vi "ScurrDataOut.vi"(8 "error in (no error)":errorcluster, 10 "测试类型":string, 11 "通道":u16(ring) items=["直流CH1", "直流CH2", "直流CH3", "直流CH4", "直流CH5", "直流CH6", "直流CH7", "直流CH8", ""]) -> (0 "error out 2":errorcluster, 3 "表格控件":string[][](table))   [LabVIEW 2014]
uses:
  <vilib>/addons/database/Connection.llb/DB Tools Open Connec (String).vi
  <vilib>/addons/database/Connection.llb/Conn Execute.vi
  <vilib>/addons/database/Recordset.llb/Rec Fetch Recordset Data (R).vi
  <vilib>/addons/database/Recordset.llb/Rec Destroy - Connection.vi
  <vilib>/addons/database/_DB Variant To Data/Database Variant To Data.xnode
  <vilib>/addons/database/NI_Database_API.lvlib
panel:
  in  "测试类型":u16(ring) items=["温循", "高温老练", "常温拷机", "自定义测试", "单次测试", "自动测试"]
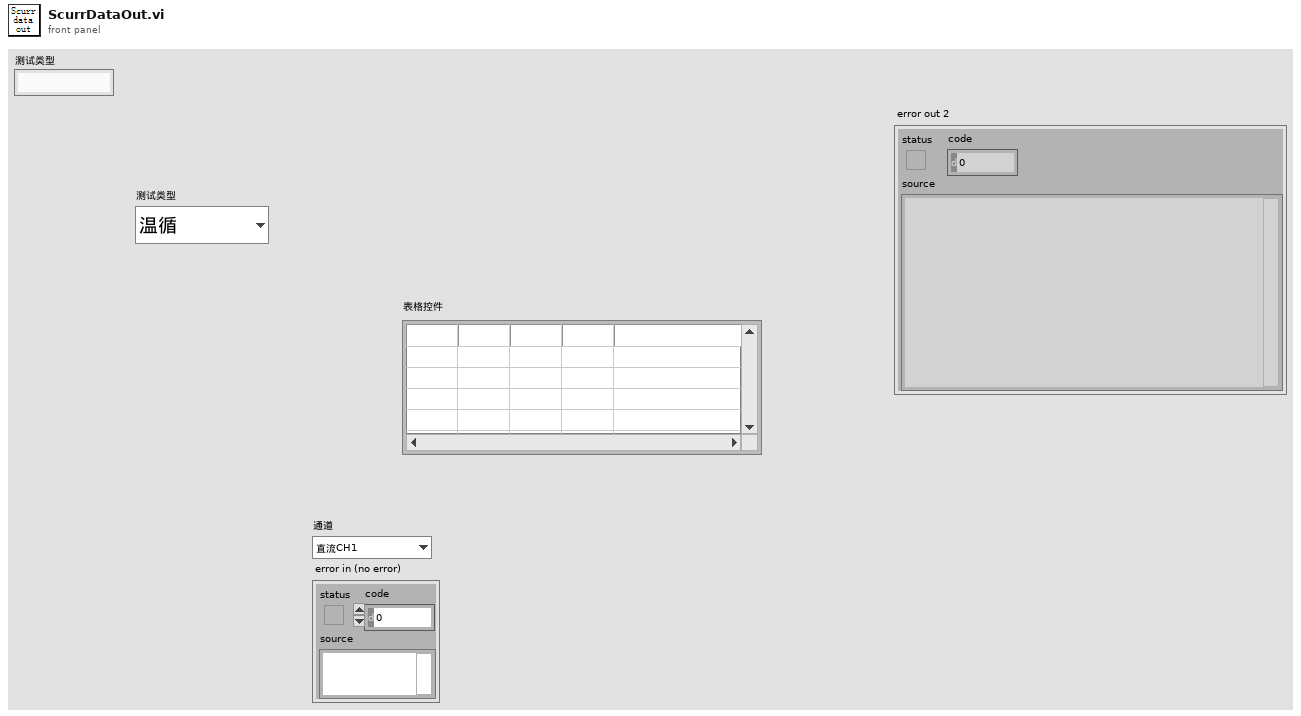
[diagram p1: front panel]
types:
  T1 = typedef "NI_Database_API.lvlib/Conn ObjectReference.ctl" = refnum<k1>
  T2 = typedef "NI_Database_API.lvlib/Rec ObjectReference.ctl" = refnum<k1>
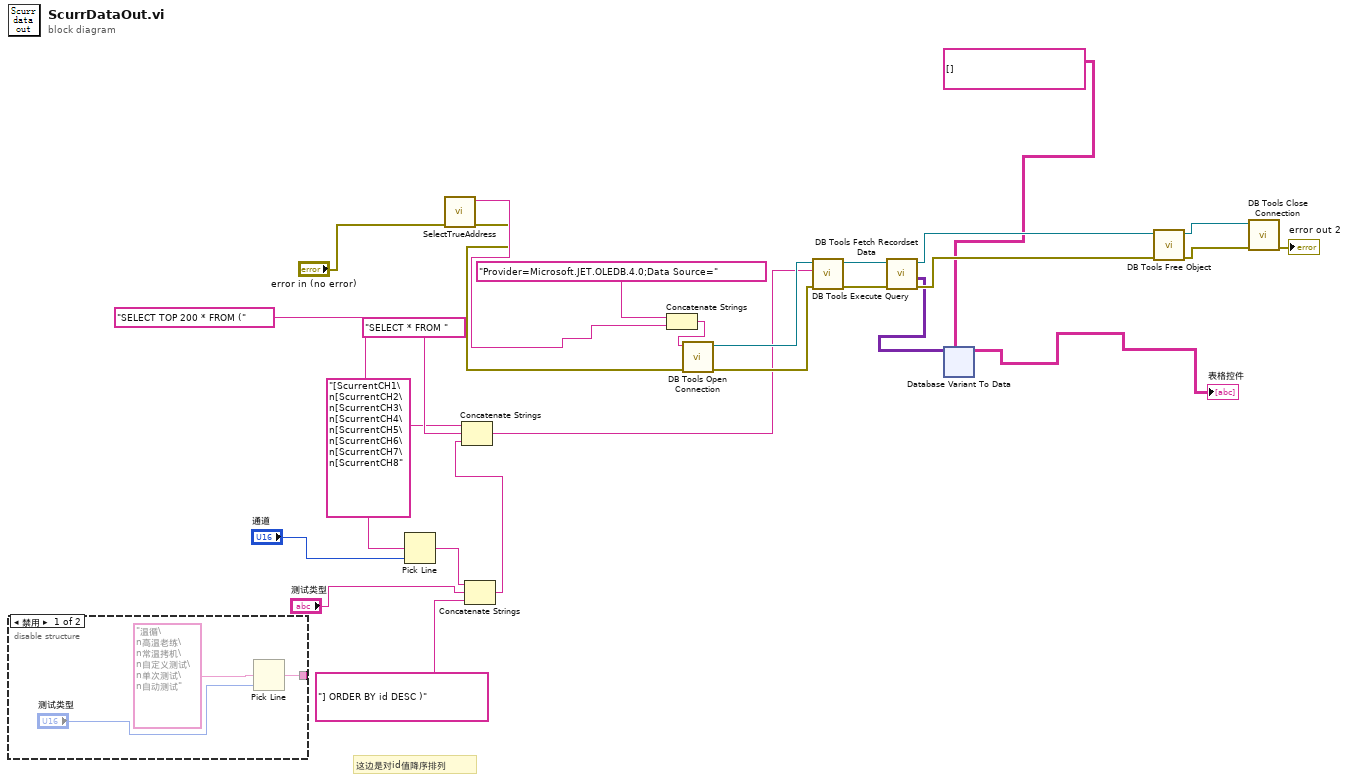
[diagram p0: block diagram]
diagram:
  # "这边是对id值降序排列"
  n1 = disable-structure shown="禁用" {
    disable-tunnel: [w27 _] -> _
    frame Disabled {
      n2 = Pick Line(multi-line string="温循\n高温老练\n常温拷机\n自定义测试\n单次测试\n自动测试" ("多行字符串"), line index="测试类型") -> (output string=w27:string)  [unwired: 1 in]
    }
    frame Enabled {
    }
  }
  n3 = Pick Line(multi-line string="[ScurrentCH1\n[ScurrentCH2\n[ScurrentCH3\n[ScurrentCH4\n[ScurrentCH5\n[ScurrentCH6\n[ScurrentCH7\n[ScurrentCH8" ("多行字符串"), line index="通道") -> (output string=w3:string)  [unwired: 1 in]
  n4 = call "SelectTrueAddress.vi"("error in (no error)"="error in (no error)") -> ("error out"=w9:errorcluster, "元素"=w11:string)  [unwired: 9 in]
  n5 = Concatenate Strings(w3, "测试类型", "] ORDER BY id DESC )") -> (w21:string)
  n6 = Concatenate Strings("SELECT TOP 200 * FROM (" ("字符串"), "SELECT * FROM ", w21) -> (w6:string)
  n7 = Concatenate Strings("Provider=Microsoft.JET.OLEDB.4.0;Data Source=", w11) -> (w10:string)
  n8 = call-poly <vilib>:"DB Tools Open Connection.vi"("error in (no error)"=w9, "connection information"=w10) -> ("error out"=w7:errorcluster, "connection reference"=w8:T1)  [unwired: 6 in]
  n9 = call-poly <vilib>:"DB Tools Execute Query.vi"("error in (no error)"=w7, "SQL query"=w6, "connection reference"=w8) -> ("error out"=w16:errorcluster, "recordset reference"=w17:T2)  [unwired: 5 in]
  n10 = call-poly <vilib>:"DB Tools Fetch Recordset Data.vi"("error in (no error)"=w16, "recordset reference"=w17) -> ("error out"=w14:errorcluster, "recordset data"=w5:variant[][], "recordset reference out"=w15:T2)  [unwired: 3 in]
  n11 = xnode "Database Variant To Data"("database variant"=w5, "type"=string[][] []) -> ("data"=→"表格控件":string[][])  [unwired: 1 in, 1 out]
  n12 = call-poly <vilib>:"DB Tools Free Object.vi"("error in (no error)"=w14, "recordset reference"=w15) -> ("error out"=w19:errorcluster, "connection reference"=w18:T1)  [unwired: 8 in]
  n13 = call <vilib>:"DB Tools Close Connection.vi"("error in (no error)"=w19, "connection reference"=w18) -> ("error out"=→"error out 2":errorcluster)  [unwired: 5 in]
